vi "ProfilerTest.vi"() -> ()   [LabVIEW 2014] (continued)
"delVelocity"=-0.7071067811865339}, {"Time"=3.0799999999999783, "delVelocity"=-0.7071067811865339}, {"Time"=3.089999999999978, "delVelocity"=-0.7071067811865311}, {"Time"=3.099999999999978, "delVelocity"=-0.7071067811865311}, {"Time"=3.1099999999999777, "delVelocity"=-0.7071067811865339}, {"Time"=3.1199999999999775, "delVelocity"=-0.7071067811865339}, {"Time"=3.1299999999999772, "delVelocity"=-0.7071067811865311}, {"Time"=3.139999999999977, "delVelocity"=-0.7071067811865311}, {"Time"=3.149999999999977, "delVelocity"=-0.7071067811865339}, {"Time"=3.1599999999999766, "delVelocity"=-0.7071067811865311}, {"Time"=3.1699999999999764, "delVelocity"=-0.7071067811865325}, {"Time"=3.179999999999976, "delVelocity"=-0.7070728008063617}, {"Time"=3.189999999999976, "delVelocity"=-0.7071407609266486}, {"Time"=3.1999999999999758, "delVelocity"=-0.7070510609334681}, {"Time"=3.2099999999999755, "delVelocity"=-0.7063739432691715}, {"Time"=3.2199999999999753, "delVelocity"=-0.7040893691122082}, {"Time"=3.229999999999975, "delVelocity"=-0.6992484530265658}, {"Time"=3.239999999999975, "delVelocity"=-0.6910154649764799}, {"Time"=3.2499999999999747, "delVelocity"=-0.6787048235649518}, {"Time"=3.2599999999999745, "delVelocity"=-0.6618114430059288}, {"Time"=3.2699999999999743, "delVelocity"=-0.6400330905341769}, {"Time"=3.279999999999974, "delVelocity"=-0.6132837646115059}, {"Time"=3.289999999999974, "delVelocity"=-0.5816975017486937}, {"Time"=3.2999999999999736, "delVelocity"=-0.5456224434357088}, {"Time"=3.3099999999999734, "delVelocity"=-0.5056054258050918}, {"Time"=3.319999999999973, "delVelocity"=-0.46236777416054364}, {"Time"=3.329999999999973, "delVelocity"=-0.41677337381576807}, {"Time"=3.3399999999999728, "delVelocity"=-0.3697904305744154}, {"Time"=3.3499999999999726, "delVelocity"=-0.322448613507402}, {"Time"=3.3599999999999723, "delVelocity"=-0.27579347708461266}, {"Time"=3.369999999999972, "delVelocity"=-0.23084018014602886}, {"Time"=3.379999999999972, "delVelocity"=-0.1885285503226669}, {"Time"=3.3899999999999717, "delVelocity"=-0.1496814829618165}, {"Time"=3.3999999999999715, "delVelocity"=-0.11496851601058011}, {"Time"=3.4099999999999713, "delVelocity"=-0.08487619320028256}, {"Time"=3.419999999999971, "delVelocity"=-0.05968652739282432}, {"Time"=3.429999999999971, "delVelocity"=-0.039464517400002175}, {"Time"=3.4399999999999706, "delVelocity"=-0.024055270838406473}, {"Time"=3.4499999999999704, "delVelocity"=-0.01309086037564744}, {"Time"=3.45999999999997, "delVelocity"=-0.006006609878955738}, {"Time"=3.46999999999997, "delVelocity"=-0.0020660895667198864}, {"Time"=3.47999999999997, "delVelocity"=-0.00039371376296115645}, {"Time"=3.4899999999999696, "delVelocity"=0.0}, {"Time"=3.4999999999999694, "delVelocity"=0.0}, {"Time"=3.509999999999969, "delVelocity"=0.0}, {"Time"=3.519999999999969, "delVelocity"=0.0}, {"Time"=3.5299999999999687, "delVelocity"=0.0}, {"Time"=3.5399999999999685, "delVelocity"=0.0}, {"Time"=3.5499999999999683, "delVelocity"=0.0}, {"Time"=3.559999999999968, "delVelocity"=0.0}, {"Time"=3.569999999999968, "delVelocity"=0.0}, {"Time"=3.5799999999999677, "delVelocity"=0.0}, {"Time"=3.5899999999999674, "delVelocity"=0.0}, {"Time"=3.5999999999999672, "delVelocity"=0.0}, {"Time"=3.609999999999967, "delVelocity"=0.0}, {"Time"=3.619999999999967, "delVelocity"=0.0}, {"Time"=3.6299999999999666, "delVelocity"=0.0}, {"Time"=3.6399999999999664, "delVelocity"=0.0}, {"Time"=3.649999999999966, "delVelocity"=0.0}, {"Time"=3.659999999999966, "delVelocity"=0.0}, {"Time"=3.6699999999999657, "delVelocity"=0.0}, {"Time"=3.6799999999999655, "delVelocity"=0.0}, {"Time"=3.6899999999999653, "delVelocity"=0.0}, {"Time"=3.699999999999965, "delVelocity"=0.0}, {"Time"=3.709999999999965, "delVelocity"=0.0}, {"Time"=3.7199999999999647, "delVelocity"=0.0}, {"Time"=3.7299999999999645, "delVelocity"=0.0}, {"Time"=3.7399999999999642, "delVelocity"=0.0}, {"Time"=3.749999999999964, "delVelocity"=0.0}, {"Time"=3.759999999999964, "delVelocity"=0.0}, {"Time"=3.7699999999999636, "delVelocity"=0.0}, {"Time"=3.7799999999999634, "delVelocity"=0.0}, {"Time"=3.789999999999963, "delVelocity"=0.0}, {"Time"=3.799999999999963, "delVelocity"=0.0}, {"Time"=3.8099999999999627, "delVelocity"=0.0}, {"Time"=3.8199999999999625, "delVelocity"=0.0}, {"Time"=3.8299999999999623, "delVelocity"=0.0}, {"Time"=3.839999999999962, "delVelocity"=0.0}, {"Time"=3.849999999999962, "delVelocity"=0.0}, {"Time"=3.8599999999999617, "delVelocity"=0.0}, {"Time"=3.8699999999999615, "delVelocity"=0.0}, {"Time"=3.8799999999999613, "delVelocity"=0.0}, {"Time"=3.889999999999961, "delVelocity"=0.0}, {"Time"=3.899999999999961, "delVelocity"=0.0}, {"Time"=3.9099999999999606, "delVelocity"=0.0}, {"Time"=3.9199999999999604, "delVelocity"=0.0}, {"Time"=3.92999999999996, "delVelocity"=0.0}, {"Time"=3.93999999999996, "delVelocity"=0.0}, {"Time"=3.9499999999999598, "delVelocity"=0.0}, {"Time"=3.9599999999999596, "delVelocity"=0.0}, {"Time"=3.9699999999999593, "delVelocity"=0.0}, {"Time"=3.979999999999959, "delVelocity"=0.0}, {"Time"=3.989999999999959, "delVelocity"=0.0}, {"Time"=3.9999999999999587, "delVelocity"=0.0}, {"Time"=4.009999999999959, "delVelocity"=0.0}, {"Time"=4.019999999999959, "delVelocity"=0.0}, {"Time"=4.0299999999999585, "delVelocity"=0.0}, {"Time"=4.039999999999958, "delVelocity"=0.0}, {"Time"=4.049999999999958, "delVelocity"=0.0}, {"Time"=4.059999999999958, "delVelocity"=0.0}, {"Time"=4.069999999999958, "delVelocity"=0.0}, {"Time"=4.079999999999957, "delVelocity"=0.0}, {"Time"=4.089999999999957, "delVelocity"=0.0}, {"Time"=4.099999999999957, "delVelocity"=0.0}, {"Time"=4.109999999999957, "delVelocity"=0.0}, {"Time"=4.119999999999957, "delVelocity"=0.0}, {"Time"=4.129999999999956, "delVelocity"=0.0}, {"Time"=4.139999999999956, "delVelocity"=0.0}, {"Time"=4.149999999999956, "delVelocity"=0.0}, {"Time"=4.159999999999956, "delVelocity"=0.0}, {"Time"=4.1699999999999555, "delVelocity"=0.0}, {"Time"=4.179999999999955, "delVelocity"=0.0}, {"Time"=4.189999999999955, "delVelocity"=0.0}, {"Time"=4.199999999999955, "delVelocity"=0.0}, {"Time"=4.209999999999955, "delVelocity"=0.0}, {"Time"=4.2199999999999545, "delVelocity"=0.0}, {"Time"=4.229999999999954, "delVelocity"=0.0}, {"Time"=4.239999999999954, "delVelocity"=0.0}, {"Time"=4.249999999999954, "delVelocity"=0.0}, {"Time"=4.259999999999954, "delVelocity"=0.0}, {"Time"=4.269999999999953, "delVelocity"=0.0}, {"Time"=4.279999999999953, "delVelocity"=0.0}, {"Time"=4.289999999999953, "delVelocity"=0.0}, {"Time"=4.299999999999953, "delVelocity"=0.0}, {"Time"=4.3099999999999525, "delVelocity"=0.0}, {"Time"=4.319999999999952, "delVelocity"=0.0}, {"Time"=4.329999999999952, "delVelocity"=0.0}, {"Time"=4.339999999999952, "delVelocity"=0.0}, {"Time"=4.349999999999952, "delVelocity"=0.0}, {"Time"=4.3599999999999515, "delVelocity"=0.0}, {"Time"=4.369999999999951, "delVelocity"=0.0}, {"Time"=4.379999999999951, "delVelocity"=0.0}, {"Time"=4.389999999999951, "delVelocity"=0.0}, {"Time"=4.399999999999951, "delVelocity"=0.0}, {"Time"=4.40999999999995, "delVelocity"=0.0}, {"Time"=4.41999999999995, "delVelocity"=0.0}, {"Time"=4.42999999999995, "delVelocity"=0.0}, {"Time"=4.43999999999995, "delVelocity"=0.0}, {"Time"=4.4499999999999496, "delVelocity"=0.0}, {"Time"=4.459999999999949, "delVelocity"=0.0}, {"Time"=4.469999999999949, "delVelocity"=0.0}, {"Time"=4.479999999999949, "delVelocity"=0.0}, {"Time"=4.489999999999949, "delVelocity"=0.0}, {"Time"=4.4999999999999485, "delVelocity"=0.0}, {"Time"=4.509999999999948, "delVelocity"=0.0}, {"Time"=4.519999999999948, "delVelocity"=0.0}, {"Time"=4.529999999999948, "delVelocity"=0.0}, {"Time"=4.539999999999948, "delVelocity"=0.0}, {"Time"=4.549999999999947, "delVelocity"=0.0}, {"Time"=4.559999999999947, "delVelocity"=0.0}, {"Time"=4.569999999999947, "delVelocity"=0.0}, {"Time"=4.579999999999947, "delVelocity"=0.0}, {"Time"=4.589999999999947, "delVelocity"=0.0}, {"Time"=4.599999999999946, "delVelocity"=0.0}, {"Time"=4.609999999999946, "delVelocity"=0.0}, {"Time"=4.619999999999946, "delVelocity"=0.0}, {"Time"=4.629999999999946, "delVelocity"=0.0}, {"Time"=4.6399999999999455, "delVelocity"=0.0}, {"Time"=4.649999999999945, "delVelocity"=0.0}, {"Time"=4.659999999999945, "delVelocity"=0.0}, {"Time"=4.669999999999945, "delVelocity"=0.0}, {"Time"=4.679999999999945, "delVelocity"=0.0}, {"Time"=4.689999999999944, "delVelocity"=0.0}, {"Time"=4.699999999999944, "delVelocity"=0.0}, {"Time"=4.709999999999944, "delVelocity"=0.0}, {"Time"=4.719999999999944, "delVelocity"=0.0}, {"Time"=4.729999999999944, "delVelocity"=0.0}, {"Time"=4.739999999999943, "delVelocity"=0.0}, {"Time"=4.749999999999943, "delVelocity"=0.0}, {"Time"=4.759999999999943, "delVelocity"=0.0}, {"Time"=4.769999999999943, "delVelocity"=0.0}, {"Time"=4.7799999999999425, "delVelocity"=0.0}, {"Time"=4.789999999999942, "delVelocity"=0.0}, {"Time"=4.799999999999942, "delVelocity"=0.0}, {"Time"=4.809999999999942, "delVelocity"=0.0}, {"Time"=4.819999999999942, "delVelocity"=0.0}, {"Time"=4.8299999999999415, "delVelocity"=0.0}, {"Time"=4.839999999999941, "delVelocity"=0.0}, {"Time"=4.849999999999941, "delVelocity"=0.0}, {"Time"=4.859999999999941, "delVelocity"=0.0}, {"Time"=4.869999999999941, "delVelocity"=0.0}, {"Time"=4.87999999999994, "delVelocity"=0.0}, {"Time"=4.88999999999994, "delVelocity"=0.0}, {"Time"=4.89999999999994, "delVelocity"=0.0}, {"Time"=4.90999999999994, "delVelocity"=0.0}, {"Time"=4.9199999999999395, "delVelocity"=0.0}, {"Time"=4.929999999999939, "delVelocity"=0.0}, {"Time"=4.939999999999939, "delVelocity"=0.0}, {"Time"=4.949999999999939, "delVelocity"=0.0}, {"Time"=4.959999999999939, "delVelocity"=0.0}, {"Time"=4.9699999999999385, "delVelocity"=0.0}, {"Time"=4.979999999999938, "delVelocity"=0.0}, {"Time"=4.989999999999938, "delVelocity"=0.0}, {"Time"=4.999999999999938, "delVelocity"=0.0}, {"Time"=5.009999999999938, "delVelocity"=0.0}, {"Time"=5.019999999999937, "delVelocity"=0.0}, {"Time"=5.029999999999937, "delVelocity"=0.0}, {"Time"=5.039999999999937, "delVelocity"=0.0}, {"Time"=5.049999999999937, "delVelocity"=0.0}, {"Time"=5.0599999999999365, "delVelocity"=0.0}, {"Time"=5.069999999999936, "delVelocity"=0.0}, {"Time"=5.079999999999936, "delVelocity"=0.0}, {"Time"=5.089999999999936, "delVelocity"=0.0}, {"Time"=5.099999999999936, "delVelocity"=0.0}, {"Time"=5.1099999999999355, "delVelocity"=0.0}, {"Time"=5.119999999999935, "delVelocity"=0.0}, {"Time"=5.129999999999935, "delVelocity"=0.0}, {"Time"=5.139999999999935, "delVelocity"=0.0}, {"Time"=5.149999999999935, "delVelocity"=0.0}, {"Time"=5.159999999999934, "delVelocity"=0.0}, {"Time"=5.169999999999934, "delVelocity"=0.0}, {"Time"=5.179999999999934, "delVelocity"=0.0}, {"Time"=5.189999999999934, "delVelocity"=0.0}, {"Time"=5.199999999999934, "delVelocity"=0.0}, {"Time"=5.209999999999933, "delVelocity"=0.0}, {"Time"=5.219999999999933, "delVelocity"=0.0}, {"Time"=5.229999999999933, "delVelocity"=0.0}, {"Time"=5.239999999999933, "delVelocity"=0.0}, {"Time"=5.2499999999999325, "delVelocity"=0.0}, {"Time"=5.259999999999932, "delVelocity"=0.0}, {"Time"=5.269999999999932, "delVelocity"=0.0}, {"Time"=5.279999999999932, "delVelocity"=0.0}, {"Time"=5.289999999999932, "delVelocity"=0.0}, {"Time"=5.299999999999931, "delVelocity"=0.0}, {"Time"=5.309999999999931, "delVelocity"=0.0}, {"Time"=5.319999999999931, "delVelocity"=0.0}, {"Time"=5.329999999999931, "delVelocity"=0.0}, {"Time"=5.339999999999931, "delVelocity"=0.0}, {"Time"=5.34999999999993, "delVelocity"=0.0}, {"Time"=5.35999999999993, "delVelocity"=0.0}, {"Time"=5.36999999999993, "delVelocity"=0.0}, {"Time"=5.37999999999993, "delVelocity"=0.0}, {"Time"=5.3899999999999295, "delVelocity"=0.0}, {"Time"=5.399999999999929, "delVelocity"=0.0}, {"Time"=5.409999999999929, "delVelocity"=0.0}, {"Time"=5.419999999999929, "delVelocity"=0.0}, {"Time"=5.429999999999929, "delVelocity"=0.0}, {"Time"=5.4399999999999284, "delVelocity"=0.0}, {"Time"=5.449999999999928, "delVelocity"=0.0}, {"Time"=5.459999999999928, "delVelocity"=0.0}, {"Time"=5.469999999999928, "delVelocity"=0.0}, {"Time"=5.479999999999928, "delVelocity"=0.0}, {"Time"=5.489999999999927, "delVelocity"=0.0}, {"Time"=5.499999999999927, "delVelocity"=0.0}, {"Time"=5.509999999999927, "delVelocity"=0.0}, {"Time"=5.519999999999927, "delVelocity"=0.0}, {"Time"=5.5299999999999265, "delVelocity"=0.0}, {"Time"=5.539999999999926, "delVelocity"=0.0}, {"Time"=5.549999999999926, "delVelocity"=0.0}, {"Time"=5.559999999999926, "delVelocity"=0.0}, {"Time"=5.569999999999926, "delVelocity"=0.0}, {"Time"=5.5799999999999255, "delVelocity"=0.0}, {"Time"=5.589999999999925, "delVelocity"=0.0}, {"Time"=5.599999999999925, "delVelocity"=0.0}, {"Time"=5.609999999999925, "delVelocity"=0.0}, {"Time"=5.619999999999925, "delVelocity"=0.0}, {"Time"=5.629999999999924, "delVelocity"=0.0}, {"Time"=5.639999999999924, "delVelocity"=0.0}, {"Time"=5.649999999999924, "delVelocity"=0.0}, {"Time"=5.659999999999924, "delVelocity"=0.0}, {"Time"=5.6699999999999235, "delVelocity"=0.0}, {"Time"=5.679999999999923, "delVelocity"=0.0}, {"Time"=5.689999999999923, "delVelocity"=0.0}, {"Time"=5.699999999999923, "delVelocity"=0.0}, {"Time"=5.709999999999923, "delVelocity"=0.0}, {"Time"=5.7199999999999225, "delVelocity"=0.0}, {"Time"=5.729999999999922, "delVelocity"=0.0}, {"Time"=5.739999999999922, "delVelocity"=0.0}, {"Time"=5.749999999999922, "delVelocity"=0.0}, {"Time"=5.759999999999922, "delVelocity"=0.0}, {"Time"=5.769999999999921, "delVelocity"=0.0}, {"Time"=5.779999999999921, "delVelocity"=0.0}, {"Time"=5.789999999999921, "delVelocity"=0.0}, {"Time"=5.799999999999921, "delVelocity"=0.0}, {"Time"=5.809999999999921, "delVelocity"=0.0}, {"Time"=5.81999999999992, "delVelocity"=0.0}, {"Time"=5.82999999999992, "delVelocity"=0.0}, {"Time"=5.83999999999992, "delVelocity"=0.0}, {"Time"=5.84999999999992, "delVelocity"=0.0}, {"Time"=5.8599999999999195, "delVelocity"=0.0}, {"Time"=5.869999999999919, "delVelocity"=0.0}, {"Time"=5.879999999999919, "delVelocity"=0.0}, {"Time"=5.889999999999919, "delVelocity"=0.0}, {"Time"=5.899999999999919, "delVelocity"=0.0}, {"Time"=5.909999999999918, "delVelocity"=0.0}, {"Time"=5.919999999999918, "delVelocity"=0.0}, {"Time"=5.929999999999918, "delVelocity"=0.0}, {"Time"=5.939999999999918, "delVelocity"=0.0}, {"Time"=5.949999999999918, "delVelocity"=0.0}, {"Time"=5.959999999999917, "delVelocity"=0.0}, {"Time"=5.969999999999917, "delVelocity"=0.0}, {"Time"=5.979999999999917, "delVelocity"=0.0}, {"Time"=5.989999999999917, "delVelocity"=0.0}, {"Time"=5.9999999999999165, "delVelocity"=0.0}, {"Time"=6.009999999999916, "delVelocity"=0.0}, {"Time"=6.019999999999916, "delVelocity"=0.0}, {"Time"=6.029999999999916, "delVelocity"=0.0}, {"Time"=6.039999999999916, "delVelocity"=0.0}, {"Time"=6.0499999999999154, "delVelocity"=0.0}, {"Time"=6.059999999999915, "delVelocity"=0.0}, {"Time"=6.069999999999915, "delVelocity"=0.0}, {"Time"=6.079999999999915, "delVelocity"=0.0}, {"Time"=6.089999999999915, "delVelocity"=0.0}, {"Time"=6.099999999999914, "delVelocity"=0.0}, {"Time"=6.109999999999914, "delVelocity"=0.0}, {"Time"=6.119999999999914, "delVelocity"=0.0}, {"Time"=6.129999999999914, "delVelocity"=0.0}, {"Time"=6.1399999999999135, "delVelocity"=0.0}, {"Time"=6.149999999999913, "delVelocity"=0.0}, {"Time"=6.159999999999913, "delVelocity"=0.0}, {"Time"=6.169999999999913, "delVelocity"=0.0}, {"Time"=6.179999999999913, "delVelocity"=0.0}, {"Time"=6.1899999999999125, "delVelocity"=0.0}, {"Time"=6.199999999999912, "delVelocity"=0.0}, {"Time"=6.209999999999912, "delVelocity"=0.0}, {"Time"=6.219999999999912, "delVelocity"=0.0}, {"Time"=6.229999999999912, "delVelocity"=0.0}, {"Time"=6.239999999999911, "delVelocity"=0.0}, {"Time"=6.249999999999911, "delVelocity"=0.0}, {"Time"=6.259999999999911, "delVelocity"=0.0}, {"Time"=6.269999999999911, "delVelocity"=0.0}, {"Time"=6.2799999999999105, "delVelocity"=0.0}, {"Time"=6.28999999999991, "delVelocity"=0.0}, {"Time"=6.29999999999991, "delVelocity"=0.0}, {"Time"=6.30999999999991, "delVelocity"=0.0}, {"Time"=6.31999999999991, "delVelocity"=0.0}, {"Time"=6.3299999999999095, "delVelocity"=0.0}, {"Time"=6.339999999999909, "delVelocity"=0.0}, {"Time"=6.349999999999909, "delVelocity"=0.0}, {"Time"=6.359999999999909, "delVelocity"=0.0}, {"Time"=6.369999999999909, "delVelocity"=0.0}, {"Time"=6.379999999999908, "delVelocity"=0.0}, {"Time"=6.389999999999908, "delVelocity"=0.0}, {"Time"=6.399999999999908, "delVelocity"=0.0}, {"Time"=6.409999999999908, "delVelocity"=0.0}, {"Time"=6.419999999999908, "delVelocity"=0.0}, {"Time"=6.429999999999907, "delVelocity"=0.0}, {"Time"=6.439999999999907, "delVelocity"=0.0}, {"Time"=6.449999999999907, "delVelocity"=0.0}, {"Time"=6.459999999999907, "delVelocity"=0.0}, {"Time"=6.4699999999999065, "delVelocity"=0.0}, {"Time"=6.479999999999906, "delVelocity"=0.0}, {"Time"=6.489999999999906, "delVelocity"=0.0}, {"Time"=6.499999999999906, "delVelocity"=0.0}, {"Time"=6.509999999999906, "delVelocity"=0.0}, {"Time"=6.519999999999905, "delVelocity"=0.0}, {"Time"=6.529999999999905, "delVelocity"=0.0}, {"Time"=6.539999999999905, "delVelocity"=0.0}, {"Time"=6.549999999999905, "delVelocity"=0.0}, {"Time"=6.559999999999905, "delVelocity"=0.0}, {"Time"=6.569999999999904, "delVelocity"=0.0}, {"Time"=6.579999999999904, "delVelocity"=0.0}, {"Time"=6.589999999999904, "delVelocity"=0.0}, {"Time"=6.599999999999904, "delVelocity"=0.0}, {"Time"=6.6099999999999035, "delVelocity"=0.0}, {"Time"=6.619999999999903, "delVelocity"=0.0}, {"Time"=6.629999999999903, "delVelocity"=0.0}, {"Time"=6.639999999999903, "delVelocity"=0.0}, {"Time"=6.649999999999903, "delVelocity"=0.0}, {"Time"=6.659999999999902, "delVelocity"=0.0}, {"Time"=6.669999999999902, "delVelocity"=0.0}, {"Time"=6.679999999999902, "delVelocity"=0.0}, {"Time"=6.689999999999902, "delVelocity"=0.0}, {"Time"=6.699999999999902, "delVelocity"=0.0}, {"Time"=6.709999999999901, "delVelocity"=0.0}, {"Time"=6.719999999999901, "delVelocity"=0.0}, {"Time"=6.729999999999901, "delVelocity"=0.0}, {"Time"=6.739999999999901, "delVelocity"=0.0}, {"Time"=6.7499999999999005, "delVelocity"=0.0}, {"Time"=6.7599999999999, "delVelocity"=0.0}, {"Time"=6.7699999999999, "delVelocity"=0.0}, {"Time"=6.7799999999999, "delVelocity"=0.0}, {"Time"=6.7899999999999, "delVelocity"=0.0}, {"Time"=6.7999999999998995, "delVelocity"=0.0}, {"Time"=6.809999999999899, "delVelocity"=0.0}, {"Time"=6.819999999999899, "delVelocity"=0.0}, {"Time"=6.829999999999899, "delVelocity"=0.0}, {"Time"=6.839999999999899, "delVelocity"=0.0}, {"Time"=6.849999999999898, "delVelocity"=0.0}, {"Time"=6.859999999999898, "delVelocity"=0.0}, {"Time"=6.869999999999898, "delVelocity"=0.0}, {"Time"=6.879999999999898, "delVelocity"=0.0}, {"Time"=6.8899999999998975, "delVelocity"=0.0}, {"Time"=6.899999999999897, "delVelocity"=0.0}, {"Time"=6.909999999999897, "delVelocity"=0.0}, {"Time"=6.919999999999897, "delVelocity"=0.0}, {"Time"=6.929999999999897, "delVelocity"=0.0}, {"Time"=6.9399999999998965, "delVelocity"=0.0}, {"Time"=6.949999999999896, "delVelocity"=0.0}, {"Time"=6.959999999999896, "delVelocity"=0.0}, {"Time"=6.969999999999896, "delVelocity"=0.0}, {"Time"=6.979999999999896, "delVelocity"=0.0}, {"Time"=6.989999999999895, "delVelocity"=0.0}, {"Time"=6.999999999999895, "delVelocity"=0.0}, {"Time"=7.009999999999895, "delVelocity"=0.0}, {"Time"=7.019999999999895, "delVelocity"=0.0}, {"Time"=7.0299999999998946, "delVelocity"=0.0}, {"Time"=7.039999999999894, "delVelocity"=0.0}, {"Time"=7.049999999999894, "delVelocity"=0.0}, {"Time"=7.059999999999894, "delVelocity"=0.0}, {"Time"=7.069999999999894, "delVelocity"=0.0}, {"Time"=7.0799999999998935, "delVelocity"=0.0}, {"Time"=7.089999999999893, "delVelocity"=0.0}, {"Time"=7.099999999999893, "delVelocity"=0.0}, {"Time"=7.109999999999893, "delVelocity"=0.0}, {"Time"=7.119999999999893, "delVelocity"=0.0}, {"Time"=7.129999999999892, "delVelocity"=0.0}, {"Time"=7.139999999999892, "delVelocity"=0.0}, {"Time"=7.149999999999892, "delVelocity"=0.0}, {"Time"=7.159999999999892, "delVelocity"=0.0}, {"Time"=7.169999999999892, "delVelocity"=0.0}, {"Time"=7.179999999999891, "delVelocity"=0.0}, {"Time"=7.189999999999891, "delVelocity"=0.0}, {"Time"=7.199999999999891, "delVelocity"=0.0}, {"Time"=7.209999999999891, "delVelocity"=0.0}, {"Time"=7.2199999999998905, "delVelocity"=0.0}, {"Time"=7.22999999999989, "delVelocity"=0.0}, {"Time"=7.23999999999989, "delVelocity"=0.0}, {"Time"=7.24999999999989, "delVelocity"=0.0}, {"Time"=7.25999999999989, "delVelocity"=0.0}, {"Time"=7.269999999999889, "delVelocity"=0.0}, {"Time"=7.279999999999889, "delVelocity"=0.0}, {"Time"=7.289999999999889, "delVelocity"=0.0}, {"Time"=7.299999999999889, "delVelocity"=0.0}, {"Time"=7.309999999999889, "delVelocity"=0.0}, {"Time"=7.319999999999888, "delVelocity"=0.0}, {"Time"=7.329999999999888, "delVelocity"=0.0}, {"Time"=7.339999999999888, "delVelocity"=0.0}, {"Time"=7.349999999999888, "delVelocity"=0.0}, {"Time"=7.3599999999998875, "delVelocity"=0.0}, {"Time"=7.369999999999887, "delVelocity"=0.0}, {"Time"=7.379999999999887, "delVelocity"=0.0}, {"Time"=7.389999999999887, "delVelocity"=0.0}, {"Time"=7.399999999999887, "delVelocity"=0.0}, {"Time"=7.4099999999998865, "delVelocity"=0.0}, {"Time"=7.419999999999886, "delVelocity"=0.0}, {"Time"=7.429999999999886, "delVelocity"=0.0}, {"Time"=7.439999999999886, "delVelocity"=0.0}, {"Time"=7.449999999999886, "delVelocity"=0.0}, {"Time"=7.459999999999885, "delVelocity"=0.0}, {"Time"=7.469999999999885, "delVelocity"=0.0}, {"Time"=7.479999999999885, "delVelocity"=0.0}, {"Time"=7.489999999999885, "delVelocity"=0.0}, {"Time"=7.4999999999998845, "delVelocity"=0.0}, {"Time"=7.509999999999884, "delVelocity"=0.0}, {"Time"=7.519999999999884, "delVelocity"=0.0}, {"Time"=7.529999999999884, "delVelocity"=0.0}, {"Time"=7.539999999999884, "delVelocity"=0.0}, {"Time"=7.5499999999998835, "delVelocity"=0.0}, {"Time"=7.559999999999883, "delVelocity"=0.0}, {"Time"=7.569999999999883, "delVelocity"=0.0}, {"Time"=7.579999999999883, "delVelocity"=0.0}, {"Time"=7.589999999999883, "delVelocity"=0.0}, {"Time"=7.599999999999882, "delVelocity"=0.0}, {"Time"=7.609999999999882, "delVelocity"=0.0}, {"Time"=7.619999999999882, "delVelocity"=0.0}, {"Time"=7.629999999999882, "delVelocity"=0.0}, {"Time"=7.6399999999998816, "delVelocity"=0.0}, {"Time"=7.649999999999881, "delVelocity"=0.0}, {"Time"=7.659999999999881, "delVelocity"=0.0}, {"Time"=7.669999999999881, "delVelocity"=0.0}, {"Time"=7.679999999999881, "delVelocity"=0.0}, {"Time"=7.6899999999998805, "delVelocity"=0.0}, {"Time"=7.69999999999988, "delVelocity"=0.0}, {"Time"=7.70999999999988, "delVelocity"=0.0}, {"Time"=7.71999999999988, "delVelocity"=0.0}, {"Time"=7.72999999999988, "delVelocity"=0.0}, {"Time"=7.739999999999879, "delVelocity"=0.0}, {"Time"=7.749999999999879, "delVelocity"=0.0}, {"Time"=7.759999999999879, "delVelocity"=0.0}, {"Time"=7.769999999999879, "delVelocity"=0.0}, {"Time"=7.779999999999879, "delVelocity"=0.0}, {"Time"=7.789999999999878, "delVelocity"=0.0}, {"Time"=7.799999999999878, "delVelocity"=0.0}, {"Time"=7.809999999999878, "delVelocity"=0.0}, {"Time"=7.819999999999878, "delVelocity"=0.0}, {"Time"=7.8299999999998775, "delVelocity"=0.0}, {"Time"=7.839999999999877, "delVelocity"=0.0}, {"Time"=7.849999999999877, "delVelocity"=0.0}, {"Time"=7.859999999999877, "delVelocity"=0.0}, {"Time"=7.869999999999877, "delVelocity"=0.0}, {"Time"=7.879999999999876, "delVelocity"=0.0}, {"Time"=7.889999999999876, "delVelocity"=0.0}, {"Time"=7.899999999999876, "delVelocity"=0.0}, {"Time"=7.909999999999876, "delVelocity"=0.0}, {"Time"=7.919999999999876, "delVelocity"=0.0}, {"Time"=7.929999999999875, "delVelocity"=0.0}, {"Time"=7.939999999999875, "delVelocity"=0.0}, {"Time"=7.949999999999875, "delVelocity"=0.0}, {"Time"=7.959999999999875, "delVelocity"=0.0}, {"Time"=7.9699999999998745, "delVelocity"=0.0}, {"Time"=7.979999999999874, "delVelocity"=0.0}, {"Time"=7.989999999999874, "delVelocity"=0.0}, {"Time"=7.999999999999874, "delVelocity"=0.0}, {"Time"=8.009999999999874, "delVelocity"=0.0}, {"Time"=8.019999999999873, "delVelocity"=0.0}, {"Time"=8.029999999999873, "delVelocity"=0.0}, {"Time"=8.039999999999873, "delVelocity"=0.0}, {"Time"=8.049999999999873, "delVelocity"=0.0}, {"Time"=8.059999999999873, "delVelocity"=0.0}, {"Time"=8.069999999999872, "delVelocity"=0.0}, {"Time"=8.079999999999872, "delVelocity"=0.0}, {"Time"=8.089999999999872, "delVelocity"=0.0}, {"Time"=8.099999999999872, "delVelocity"=0.0}, {"Time"=8.109999999999872, "delVelocity"=0.0}, {"Time"=8.119999999999871, "delVelocity"=0.0}, {"Time"=8.129999999999871, "delVelocity"=0.0}, {"Time"=8.139999999999871, "delVelocity"=0.0}, {"Time"=8.14999999999987, "delVelocity"=0.0}, {"Time"=8.15999999999987, "delVelocity"=0.0}, {"Time"=8.16999999999987, "delVelocity"=0.0}, {"Time"=8.17999999999987, "delVelocity"=0.0}, {"Time"=8.18999999999987, "delVelocity"=0.0}, {"Time"=8.19999999999987, "delVelocity"=0.0}, {"Time"=8.20999999999987, "delVelocity"=0.0}, {"Time"=8.21999999999987, "delVelocity"=0.0}, {"Time"=8.229999999999869, "delVelocity"=0.0}, {"Time"=8.239999999999869, "delVelocity"=0.0}, {"Time"=8.249999999999869, "delVelocity"=0.0}, {"Time"=8.259999999999868, "delVelocity"=0.0}, {"Time"=8.269999999999868, "delVelocity"=0.0}, {"Time"=8.279999999999868, "delVelocity"=0.0}, {"Time"=8.289999999999868, "delVelocity"=0.0}, {"Time"=8.299999999999867, "delVelocity"=0.0}, {"Time"=8.309999999999867, "delVelocity"=0.0}, {"Time"=8.319999999999867, "delVelocity"=0.0}, {"Time"=8.329999999999867, "delVelocity"=0.0}, {"Time"=8.339999999999867, "delVelocity"=0.0}, {"Time"=8.349999999999866, "delVelocity"=0.0}, {"Time"=8.359999999999866, "delVelocity"=0.0}, {"Time"=8.369999999999866, "delVelocity"=0.0}, {"Time"=8.379999999999866, "delVelocity"=0.0}, {"Time"=8.389999999999866, "delVelocity"=0.0}, {"Time"=8.399999999999865, "delVelocity"=0.0}, {"Time"=8.409999999999865, "delVelocity"=0.0}, {"Time"=8.419999999999865, "delVelocity"=0.0}, {"Time"=8.429999999999865, "delVelocity"=0.0}, {"Time"=8.439999999999864, "delVelocity"=0.0}, {"Time"=8.449999999999864, "delVelocity"=0.0}, {"Time"=8.459999999999864, "delVelocity"=0.0}, {"Time"=8.469999999999864, "delVelocity"=0.0}, {"Time"=8.479999999999864, "delVelocity"=0.0}, {"Time"=8.489999999999863, "delVelocity"=0.0}, {"Time"=8.499999999999863, "delVelocity"=0.0}, {"Time"=8.509999999999863, "delVelocity"=0.0}, {"Time"=8.519999999999863, "delVelocity"=0.0}, {"Time"=8.529999999999863, "delVelocity"=0.0}, {"Time"=8.539999999999862, "delVelocity"=0.0}, {"Time"=8.549999999999862, "delVelocity"=0.0}, {"Time"=8.559999999999862, "delVelocity"=0.0}, {"Time"=8.569999999999862, "delVelocity"=0.0}, {"Time"=8.579999999999862, "delVelocity"=0.0}, {"Time"=8.589999999999861, "delVelocity"=0.0}, {"Time"=8.599999999999861, "delVelocity"=0.0}, {"Time"=8.60999999999986, "delVelocity"=0.0}, {"Time"=8.61999999999986, "delVelocity"=0.0}, {"Time"=8.62999999999986, "delVelocity"=0.0}, {"Time"=8.63999999999986, "delVelocity"=0.0}, {"Time"=8.64999999999986, "delVelocity"=0.0}, {"Time"=8.65999999999986, "delVelocity"=0.0}, {"Time"=8.66999999999986, "delVelocity"=0.0}, {"Time"=8.67999999999986, "delVelocity"=0.0}, {"Time"=8.68999999999986, "delVelocity"=0.0}, {"Time"=8.699999999999859, "delVelocity"=0.0}, {"Time"=8.709999999999859, "delVelocity"=0.0}, {"Time"=8.719999999999859, "delVelocity"=0.0}, {"Time"=8.729999999999858, "delVelocity"=0.0}, {"Time"=8.739999999999858, "delVelocity"=0.0}, {"Time"=8.749999999999858, "delVelocity"=0.0}, {"Time"=8.759999999999858, "delVelocity"=0.0}, {"Time"=8.769999999999857, "delVelocity"=0.0}, {"Time"=8.779999999999857, "delVelocity"=0.0}, {"Time"=8.789999999999857, "delVelocity"=0.0}, {"Time"=8.799999999999857, "delVelocity"=0.0}, {"Time"=8.809999999999857, "delVelocity"=0.0}, {"Time"=8.819999999999856, "delVelocity"=0.0}, {"Time"=8.829999999999856, "delVelocity"=0.0}, {"Time"=8.839999999999856, "delVelocity"=0.0}, {"Time"=8.849999999999856, "delVelocity"=0.0}, {"Time"=8.859999999999856, "delVelocity"=0.0}, {"Time"=8.869999999999855, "delVelocity"=0.0}, {"Time"=8.879999999999855, "delVelocity"=0.0}, {"Time"=8.889999999999855, "delVelocity"=0.0}, {"Time"=8.899999999999855, "delVelocity"=0.0}, {"Time"=8.909999999999854, "delVelocity"=0.0}, {"Time"=8.919999999999854, "delVelocity"=0.0}, {"Time"=8.929999999999854, "delVelocity"=0.0}, {"Time"=8.939999999999854, "delVelocity"=0.0}, {"Time"=8.949999999999854, "delVelocity"=0.0}, {"Time"=8.959999999999853, "delVelocity"=0.0}, {"Time"=8.969999999999853, "delVelocity"=0.0}, {"Time"=8.979999999999853, "delVelocity"=0.0}, {"Time"=8.989999999999853, "delVelocity"=0.0}, {"Time"=8.999999999999853, "delVelocity"=0.0}, {"Time"=9.009999999999852, "delVelocity"=0.0}, {"Time"=9.019999999999852, "delVelocity"=0.0}, {"Time"=9.029999999999852, "delVelocity"=0.0}, {"Time"=9.039999999999852, "delVelocity"=0.0}, {"Time"=9.049999999999851, "delVelocity"=0.0}, {"Time"=9.059999999999851, "delVelocity"=0.0}, {"Time"=9.069999999999851, "delVelocity"=0.0}, {"Time"=9.07999999999985, "delVelocity"=0.0}, {"Time"=9.08999999999985, "delVelocity"=0.0}, {"Time"=9.09999999999985, "delVelocity"=0.0}, {"Time"=9.10999999999985, "delVelocity"=0.0}, {"Time"=9.11999999999985, "delVelocity"=0.0}, {"Time"=9.12999999999985, "delVelocity"=0.0}, {"Time"=9.13999999999985, "delVelocity"=0.0}, {"Time"=9.14999999999985, "delVelocity"=0.0}, {"Time"=9.15999999999985, "delVelocity"=0.0}, {"Time"=9.169999999999849, "delVelocity"=0.0}, {"Time"=9.179999999999849, "delVelocity"=0.0}, {"Time"=9.189999999999849, "delVelocity"=0.0}, {"Time"=9.199999999999848, "delVelocity"=0.0}, {"Time"=9.209999999999848, "delVelocity"=0.0}, {"Time"=9.219999999999848, "delVelocity"=0.0}, {"Time"=9.229999999999848, "delVelocity"=0.0}, {"Time"=9.239999999999847, "delVelocity"=0.0}, {"Time"=9.249999999999847, "delVelocity"=0.0}, {"Time"=9.259999999999847, "delVelocity"=0.0}, {"Time"=9.269999999999847, "delVelocity"=0.0}, {"Time"=9.279999999999847, "delVelocity"=0.0}, {"Time"=9.289999999999846, "delVelocity"=0.0}, {"Time"=9.299999999999846, "delVelocity"=0.0}, {"Time"=9.309999999999846, "delVelocity"=0.0}, {"Time"=9.319999999999846, "delVelocity"=0.0}, {"Time"=9.329999999999846, "delVelocity"=0.0}, {"Time"=9.339999999999845, "delVelocity"=0.0}, {"Time"=9.349999999999845, "delVelocity"=0.0}, {"Time"=9.359999999999845, "delVelocity"=0.0}, {"Time"=9.369999999999845, "delVelocity"=0.0}, {"Time"=9.379999999999844, "delVelocity"=0.0}, {"Time"=9.389999999999844, "delVelocity"=0.0}, {"Time"=9.399999999999844, "delVelocity"=0.0}, {"Time"=9.409999999999844, "delVelocity"=0.0}, {"Time"=9.419999999999844, "delVelocity"=0.0}, {"Time"=9.429999999999843, "delVelocity"=0.0}, {"Time"=9.439999999999843, "delVelocity"=0.0}, {"Time"=9.449999999999843, "delVelocity"=0.0}, {"Time"=9.459999999999843, "delVelocity"=0.0}, {"Time"=9.469999999999843, "delVelocity"=0.0}, {"Time"=9.479999999999842, "delVelocity"=0.0}, {"Time"=9.489999999999842, "delVelocity"=0.0}, {"Time"=9.499999999999842, "delVelocity"=0.0}, {"Time"=9.509999999999842, "delVelocity"=0.0}, {"Time"=9.519999999999841, "delVelocity"=0.0}, {"Time"=9.529999999999841, "delVelocity"=0.0}, {"Time"=9.539999999999841, "delVelocity"=0.0}, {"Time"=9.54999999999984, "delVelocity"=0.0}, {"Time"=9.55999999999984, "delVelocity"=0.0}, {"Time"=9.56999999999984, "delVelocity"=0.0}, {"Time"=9.57999999999984, "delVelocity"=0.0}, {"Time"=9.58999999999984, "delVelocity"=0.0}, {"Time"=9.59999999999984, "delVelocity"=0.0}, {"Time"=9.60999999999984, "delVelocity"=0.0}, {"Time"=9.61999999999984, "delVelocity"=0.0}, {"Time"=9.62999999999984, "delVelocity"=0.0}, {"Time"=9.639999999999839, "delVelocity"=0.0}, {"Time"=9.649999999999839, "delVelocity"=0.0}, {"Time"=9.659999999999838, "delVelocity"=0.0}, {"Time"=9.669999999999838, "delVelocity"=0.0}, {"Time"=9.679999999999838, "delVelocity"=0.0}, {"Time"=9.689999999999838, "delVelocity"=0.0}, {"Time"=9.699999999999838, "delVelocity"=0.0}, {"Time"=9.709999999999837, "delVelocity"=0.0}, {"Time"=9.719999999999837, "delVelocity"=0.0}, {"Time"=9.729999999999837, "delVelocity"=0.0}, {"Time"=9.739999999999837, "delVelocity"=0.0}, {"Time"=9.749999999999837, "delVelocity"=0.0}, {"Time"=9.759999999999836, "delVelocity"=0.0}, {"Time"=9.769999999999836, "delVelocity"=0.0}, {"Time"=9.779999999999836, "delVelocity"=0.0}, {"Time"=9.789999999999836, "delVelocity"=0.0}, {"Time"=9.799999999999836, "delVelocity"=0.0}, {"Time"=9.809999999999835, "delVelocity"=0.0}, {"Time"=9.819999999999835, "delVelocity"=0.0}, {"Time"=9.829999999999835, "delVelocity"=0.0}, {"Time"=9.839999999999835, "delVelocity"=0.0}, {"Time"=9.849999999999834, "delVelocity"=0.0}, {"Time"=9.859999999999834, "delVelocity"=0.0}, {"Time"=9.869999999999834, "delVelocity"=0.0}, {"Time"=9.879999999999834, "delVelocity"=0.0}, {"Time"=9.889999999999834, "delVelocity"=0.0}, {"Time"=9.899999999999833, "delVelocity"=0.0}, {"Time"=9.909999999999833, "delVelocity"=0.0}, {"Time"=9.919999999999833, "delVelocity"=0.0}, {"Time"=9.929999999999833, "delVelocity"=0.0}, {"Time"=9.939999999999833, "delVelocity"=0.0}, {"Time"=9.949999999999832, "delVelocity"=0.0}, {"Time"=9.959999999999832, "delVelocity"=0.0}, {"Time"=9.969999999999832, "delVelocity"=0.0}, {"Time"=9.979999999999832, "delVelocity"=0.0}, {"Time"=9.989999999999831, "delVelocity"=0.0}, {"Time"=9.999999999999831, "delVelocity"=0.0}, {"Time"=10.009999999999831, "delVelocity"=0.0}, {"Time"=10.01999999999983, "delVelocity"=0.0}, {"Time"=10.02999999999983, "delVelocity"=0.0}, {"Time"=10.03999999999983, "delVelocity"=0.0}, {"Time"=10.04999999999983, "delVelocity"=0.0}, {"Time"=10.05999999999983, "delVelocity"=0.0}, {"Time"=10.06999999999983, "delVelocity"=0.0}, {"Time"=10.07999999999983, "delVelocity"=0.0}, {"Time"=10.08999999999983, "delVelocity"=0.0}, {"Time"=10.09999999999983, "delVelocity"=0.0}, {"Time"=10.109999999999829, "delVelocity"=0.0}, {"Time"=10.119999999999829, "delVelocity"=0.0}, {"Time"=10.129999999999828, "delVelocity"=0.0}, {"Time"=10.139999999999828, "delVelocity"=0.0}, {"Time"=10.149999999999828, "delVelocity"=0.0}, {"Time"=10.159999999999828, "delVelocity"=0.0}, {"Time"=10.169999999999828, "delVelocity"=0.0}, {"Time"=10.179999999999827, "delVelocity"=0.0}, {"Time"=10.189999999999827, "delVelocity"=0.0}, {"Time"=10.199999999999827, "delVelocity"=0.0}, {"Time"=10.209999999999827, "delVelocity"=0.0}, {"Time"=10.219999999999827, "delVelocity"=0.0}, {"Time"=10.229999999999826, "delVelocity"=0.0}, {"Time"=10.239999999999826, "delVelocity"=0.0}, {"Time"=10.249999999999826, "delVelocity"=0.0}, {"Time"=10.259999999999826, "delVelocity"=0.0}, {"Time"=10.269999999999825, "delVelocity"=0.0}, {"Time"=10.279999999999825, "delVelocity"=0.0}, {"Time"=10.289999999999825, "delVelocity"=0.0}, {"Time"=10.299999999999825, "delVelocity"=0.0}, {"Time"=10.309999999999825, "delVelocity"=0.0}, {"Time"=10.319999999999824, "delVelocity"=0.0}, {"Time"=10.329999999999824, "delVelocity"=0.0}, {"Time"=10.339999999999824, "delVelocity"=0.0}, {"Time"=10.349999999999824, "delVelocity"=0.0}, {"Time"=10.359999999999824, "delVelocity"=0.0}, {"Time"=10.369999999999823, "delVelocity"=0.0}, {"Time"=10.379999999999823, "delVelocity"=0.0}, {"Time"=10.389999999999823, "delVelocity"=0.0}, {"Time"=10.399999999999823, "delVelocity"=0.0}, {"Time"=10.409999999999823, "delVelocity"=0.0}, {"Time"=10.419999999999822, "delVelocity"=0.0}, {"Time"=10.429999999999822, "delVelocity"=0.0}, {"Time"=10.439999999999822, "delVelocity"=0.0}, {"Time"=10.449999999999822, "delVelocity"=0.0}, {"Time"=10.459999999999821, "delVelocity"=0.0}, {"Time"=10.469999999999821, "delVelocity"=0.0}, {"Time"=10.479999999999821, "delVelocity"=0.0}, {"Time"=10.48999999999982, "delVelocity"=0.0}, {"Time"=10.49999999999982, "delVelocity"=0.0}, {"Time"=10.50999999999982, "delVelocity"=0.0}, {"Time"=10.51999999999982, "delVelocity"=0.0}, {"Time"=10.52999999999982, "delVelocity"=0.0}, {"Time"=10.53999999999982, "delVelocity"=0.0}, {"Time"=10.54999999999982, "delVelocity"=0.0}, {"Time"=10.55999999999982, "delVelocity"=0.0}, {"Time"=10.569999999999819, "delVelocity"=0.0}, {"Time"=10.579999999999819, "delVelocity"=0.0}, {"Time"=10.589999999999819, "delVelocity"=0.0}, {"Time"=10.599999999999818, "delVelocity"=0.0}, {"Time"=10.609999999999818, "delVelocity"=0.0}, {"Time"=10.619999999999818, "delVelocity"=0.0}, {"Time"=10.629999999999818, "delVelocity"=0.0}, {"Time"=10.639999999999818, "delVelocity"=0.0}, {"Time"=10.649999999999817, "delVelocity"=0.0}, {"Time"=10.659999999999817, "delVelocity"=0.0}, {"Time"=10.669999999999817, "delVelocity"=0.0}, {"Time"=10.679999999999817, "delVelocity"=0.0}, {"Time"=10.689999999999817, "delVelocity"=0.0}, {"Time"=10.699999999999816, "delVelocity"=0.0}, {"Time"=10.709999999999816, "delVelocity"=0.0}, {"Time"=10.719999999999816, "delVelocity"=0.0}, {"Time"=10.729999999999816, "delVelocity"=0.0}, {"Time"=10.739999999999815, "delVelocity"=0.0}, {"Time"=10.749999999999815, "delVelocity"=0.0}, {"Time"=10.759999999999815, "delVelocity"=0.0}, {"Time"=10.769999999999815, "delVelocity"=0.0}, {"Time"=10.779999999999815, "delVelocity"=0.0}, {"Time"=10.789999999999814, "delVelocity"=0.0}, {"Time"=10.799999999999814, "delVelocity"=0.0}, {"Time"=10.809999999999814, "delVelocity"=0.0}, {"Time"=10.819999999999814, "delVelocity"=0.0}, {"Time"=10.829999999999814, "delVelocity"=0.0}, {"Time"=10.839999999999813, "delVelocity"=0.0}, {"Time"=10.849999999999813, "delVelocity"=0.0}, {"Time"=10.859999999999813, "delVelocity"=0.0}, {"Time"=10.869999999999813, "delVelocity"=0.0}, {"Time"=10.879999999999812, "delVelocity"=0.0}, {"Time"=10.889999999999812, "delVelocity"=0.0}, {"Time"=10.899999999999812, "delVelocity"=0.0}, {"Time"=10.909999999999812, "delVelocity"=0.0}, {"Time"=10.919999999999812, "delVelocity"=0.0}, {"Time"=10.929999999999811, "delVelocity"=0.0}, {"Time"=10.939999999999811, "delVelocity"=0.0}, {"Time"=10.949999999999811, "delVelocity"=0.0}, {"Time"=10.95999999999981, "delVelocity"=0.0}, {"Time"=10.96999999999981, "delVelocity"=0.0}, {"Time"=10.97999999999981, "delVelocity"=0.0}, {"Time"=10.98999999999981, "delVelocity"=0.0}, {"Time"=10.99999999999981, "delVelocity"=0.0}, {"Time"=11.00999999999981, "delVelocity"=0.0}, {"Time"=11.01999999999981, "delVelocity"=0.0}, {"Time"=11.02999999999981, "delVelocity"=0.0}, {"Time"=11.039999999999809, "delVelocity"=0.0}, {"Time"=11.049999999999809, "delVelocity"=0.0}, {"Time"=11.059999999999809, "delVelocity"=0.0}, {"Time"=11.069999999999808, "delVelocity"=0.0}, {"Time"=11.079999999999808, "delVelocity"=0.0}, {"Time"=11.089999999999808, "delVelocity"=0.0}, {"Time"=11.099999999999808, "delVelocity"=0.0}, {"Time"=11.109999999999808, "delVelocity"=0.0}, {"Time"=11.119999999999807, "delVelocity"=0.0}, {"Time"=11.129999999999807, "delVelocity"=0.0}, {"Time"=11.139999999999807, "delVelocity"=0.0}, {"Time"=11.149999999999807, "delVelocity"=0.0}, {"Time"=11.159999999999807, "delVelocity"=0.0}, {"Time"=11.169999999999806, "delVelocity"=0.0}, {"Time"=11.179999999999806, "delVelocity"=0.0}, {"Time"=11.189999999999806, "delVelocity"=0.0}, {"Time"=11.199999999999806, "delVelocity"=0.0}, {"Time"=11.209999999999805, "delVelocity"=0.0}, {"Time"=11.219999999999805, "delVelocity"=0.0}, {"Time"=11.229999999999805, "delVelocity"=0.0}, {"Time"=11.239999999999805, "delVelocity"=0.0}, {"Time"=11.249999999999805, "delVelocity"=0.0}, {"Time"=11.259999999999804, "delVelocity"=0.0}, {"Time"=11.269999999999804, "delVelocity"=0.0}, {"Time"=11.279999999999804, "delVelocity"=0.0}, {"Time"=11.289999999999804, "delVelocity"=0.0}, {"Time"=11.299999999999804, "delVelocity"=0.0}, {"Time"=11.309999999999803, "delVelocity"=0.0}, {"Time"=11.319999999999803, "delVelocity"=0.0}, {"Time"=11.329999999999803, "delVelocity"=0.0}, {"Time"=11.339999999999803, "delVelocity"=0.0}, {"Time"=11.349999999999802, "delVelocity"=0.0}, {"Time"=11.359999999999802, "delVelocity"=0.0}, {"Time"=11.369999999999802, "delVelocity"=0.0}, {"Time"=11.379999999999802, "delVelocity"=0.0}, {"Time"=11.389999999999802, "delVelocity"=0.0}, {"Time"=11.399999999999801, 
